vi "ziExample-Module-MDS.vi"() -> ()   [LabVIEW 2018]
doc: "This examples allows to control a Zurich Instruments device via a LabOne Labview API. \nThis vi enables the multi-device synchronisation of two ZI instruments of the same family.\n\n© Zurich Instruments AG, www.zhinst.com"
uses:
  Public/Modules/ziTypeModEnum.ctl
  Public/Modules/ziModSetValueDouble.vi
  Public/Modules/ziModSetValueBinary.vi
  Public/Modules/ziModGetNodeValueString.vi
  Public/Modules/ziModGetNodeValueDouble.vi
  Zurich Instruments LabOne.lvlib
panel:
  out "Status":dbl
  out "Message":string
  in  "Slave":string="dev"
  in  "Master":string="dev"
  # "ziExample-Module-MDS.vi\nRequirements: 2xHF2\nsee block diagram for VI description"
  # "Tested Devices:\n\n- HF2\n- MFLI\n- UHF"
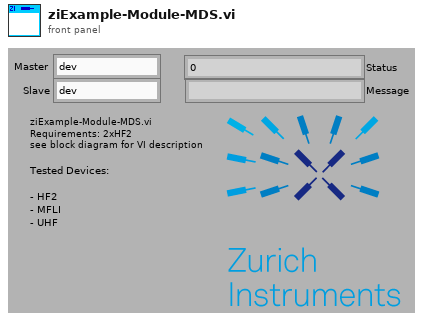
[diagram p1: front panel]
types:
  T1 = typedef "Zurich Instruments LabOne.lvlib/ziTypeModEnum.ctl" = u16
  T2 = typedef "Zurich Instruments LabOne.lvlib/ziTypeHandle.ctl" = cluster{"handleValid":bool, "Conn":u64, "Path Prefix":string, "Handle":u64, "Connected":bool, "Clockbase(s)":dbl}
  T3 = typedef "ziTypeDisovery.ctl" = cluster{"timestamp":u64, "deviceid":string, "devicetype":string, "serveraddress":string, "serverport":u32, "apilevel":u32, "discoverable":bool, "interface":string, "connected":string, "available":bool, "owner":string, "status":string, "options ":string, "serverversion":string}
  T4 = typedef "Zurich Instruments LabOne.lvlib/ziTypeModHandle.ctl" = cluster{"handleValid":bool, "Conn":u64, "ModHandle":u64, "moduleID":string, "Path Prefix":string}
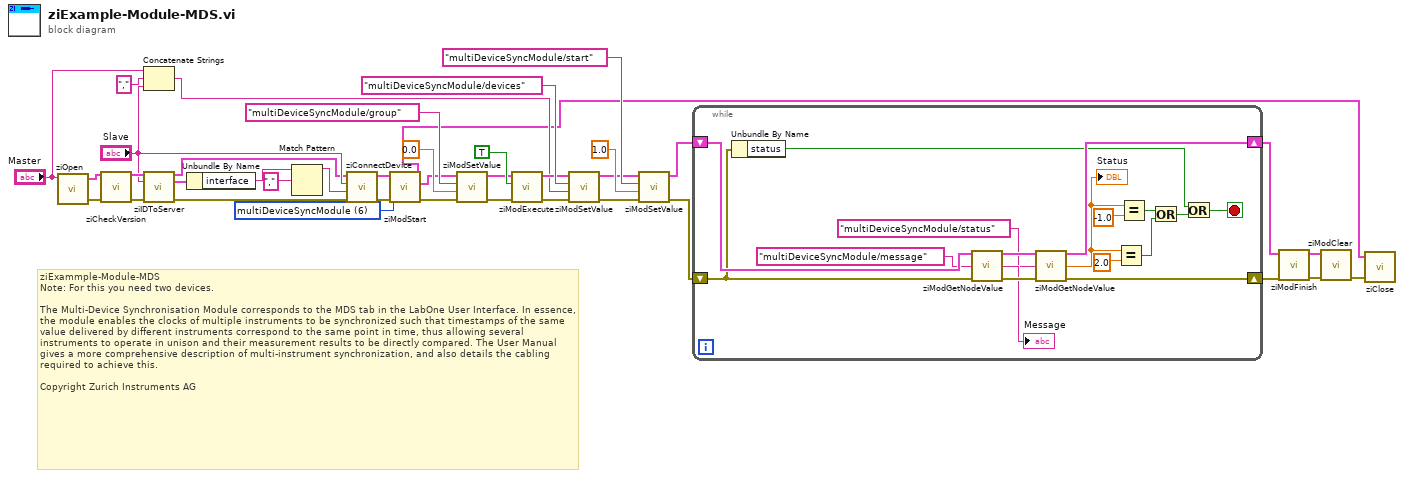
[diagram p0: block diagram]
diagram:
  w12 = T1 6 items=["sweep", "scopeModule", "dataAcquisitionModule", "pidAdvisor", "awgModule", "impedanceModule", "multiDeviceSyncModule", "zoomFFT", "trigger", "deviceSettings", "record"] ("module Id")
  # "ziExammple-Module-MDS\nNote: For this you need two devices.\n \nThe Multi-Device Synchronisation Module corresponds to the MDS tab in the LabOne User Interface. In essence, the module enables the clocks of multiple instruments to be synchronized such that timestamps of the same value delivered by different instruments correspond to the same point in time, thus allowing several instruments to operate in unison and their measurement results to be directly compared. The User Manual gives a more comprehensive description of multi-instrument synchronization, and also details the cabling required to achieve this.\n\nCopyright Zurich Instruments AG"
  n1 = call "ziOpen.vi"("Address"="Master") -> ("Error Out"=w10:errorcluster, "HandleOut"=w11:T2)  [unwired: 3 in, 1 out]
  n2 = call "ziCheckVersion.vi"("Handle In"=w11, "Error In"=w10) -> ("Handle Out"=w9:T2, "Error Out"=w7:errorcluster)  [unwired: 11 in, 1 out]
  n3 = Concatenate Strings("Master", "," ("string"), "Slave") -> (w21:string)
  n4 = call "ziIDToServer.vi"("ziHandle In"=w9, "Device ID"="Slave", "Error In"=w7) -> ("ziHandle Out"=w6:T2, "ziDiscovery"=w4:T3, "Error Out"=w5:errorcluster)  [unwired: 10 in]
  n5 = Unbundle By Name(w4) -> ("interface"=w3:string)
  n6 = Match Pattern(string=w3, regular expression=",") -> (before substring=w1:string)  [unwired: 1 in, 3 out]
  n7 = call "ziConnectDevice.vi"("Error In"=w5, "Device Interface"=w1, "Device Serial"="Slave", "Handle In"=w6) -> ("Error Out"=w38:errorcluster, "Handle Out"=w39:T2)  [unwired: 6 in]
  n8 = call "ziModStart.vi"("Error In"=w38, "module Id"=w12, "Handle In"=w39) -> ("Error Out"=w29:errorcluster, "ModHandle Out"=w26:T4, "Handle Out"=w15:T2)  [unwired: 6 in]
  n9 = call-poly "ziModSetValue.vi"("Error In"=w29, "Value"=0.0, "Path"="multiDeviceSyncModule/group", "ModHandle In"=w26) -> ("Error Out"=w28:errorcluster, "ModHandle Out"=w25:T4)  [unwired: 6 in]
  n10 = call "ziModExecute.vi"("Error In"=w28, "Modal (F)"=TRUE, "ziModHandle In"=w25) -> ("Error Out"=w27:errorcluster, "ziModHandle Out"=w24:T4)  [unwired: 5 in, 1 out]
  n11 = call-poly "ziModSetValue.vi"("Error In"=w27, "Data"=w21, "Path"="multiDeviceSyncModule/devices", "ModHandle In"=w24) -> ("Error Out"=w33:errorcluster, "ModHandle Out"=w34:T4)  [unwired: 6 in]
  n12 = call-poly "ziModSetValue.vi"("Error In"=w33, "Value"=1.0, "Path"="multiDeviceSyncModule/start", "ModHandle In"=w34) -> ("Error Out"=w19:errorcluster, "ModHandle Out"=w20:T4)  [unwired: 6 in]
  n13 = while {
    shift-right: [w48] -> w13
    shift-left: w20 -> [w55]
    shift-right: [w49] -> w18
    shift-left: w19 -> [w42]
    stop <- w40 stop-if-true
    n14 = Unbundle By Name(w42) -> ("status"=w43:bool)
    n15 = call-poly "ziModGetNodeValue.vi"("ModHandle In"=w55, "Path"="multiDeviceSyncModule/message", "error in"=w42) -> ("ModHandle Out"=w54:T4, "Value"=→"Message":string, "error out"=w53:errorcluster)  [unwired: 10 in]
    n16 = call-poly "ziModGetNodeValue.vi"("ModHandle In"=w54, "Path"="multiDeviceSyncModule/status", "error in"=w53) -> ("ModHandle Out"=w48:T4, "Value"=w45:dbl, "error out"=w49:errorcluster)  [unwired: 10 in]
    "Status" <- w45
    n17 = Equal?(x=w45, y=2.0) -> (x = y?=w46:bool)
    n18 = Equal?(x=w45, y=-1.0) -> (x = y?=w47:bool)
    n19 = Or(x=w47, y=w46) -> (x .or. y?=w41:bool)
    n20 = Or(x=w43, y=w41) -> (x .or. y?=w40:bool)
  }
  n21 = call "ziModFinish.vi"("Error In"=w18, "ziModHandle In"=w13) -> ("Error Out"=w17:errorcluster, "ziModHandle Out"=w14:T4)  [unwired: 7 in]
  n22 = call "ziModClear.vi"("Error In"=w17, "ziModHandle In"=w14) -> ("Error Out"=w16:errorcluster)  [unwired: 7 in, 1 out]
  n23 = call "ziClose.vi"("Error In"=w16, "Handle In"=w15) -> ()  [unwired: 2 in, 2 out]
